vi "Agilent DMM Measure.vi"(7 "Agilent DMM":T2, 8 "error in (no error)":errorcluster, 11 "VISA Resource Name":refnum<visa-resource-name>) -> (0 "error out":errorcluster {"code" format="%.0x"}, 2 "DMM Measurement":T1 caption="This reading is allways in the base units\ni.e. V, A, Ohms, Hz, Sec, etc." format="%#_10f", 3 "dup VISA Resource Name":refnum<visa-resource-name>)   [LabVIEW 2011]
uses:
  TypeDefs/Agilent DMM Instrument Info.ctl
  DMM Measurement.ctl
  TypeDefs/Agilent DMM Trigger Source.ctl
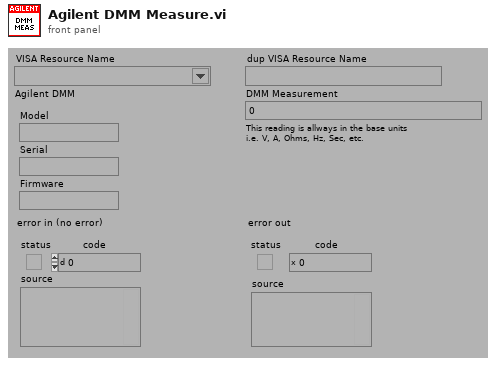
[diagram p1: front panel]
types:
  T1 = typedef "DMM Measurement.ctl" = dbl
  T2 = typedef "Agilent DMM Instrument Info.ctl" = cluster{"Model":string, "Serial":string, "Firmware":string}
  T3 = typedef "Agilent DMM Trigger Source.ctl" = enum16{"Immediate", "Bus", "External"}
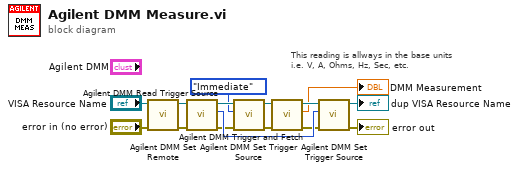
[diagram p0: block diagram]
diagram:
  # "This reading is allways in the base units\ni.e. V, A, Ohms, Hz, Sec, etc."
  n1 = call "Agilent DMM Set Remote.vi"("error in (no error)"="error in (no error)", "VISA Resource Name"="VISA Resource Name") -> ("error out"=w6:errorcluster, "dup VISA Resource Name"=w7:refnum<visa-resource-name>)  [unwired: 8 out]
  n2 = call "Agilent DMM Read Trigger Source.vi"("error in (no error)"=w6, "VISA Resource Name"=w7) -> ("error out"=w2:errorcluster, "Trigger Source"=w13:T3, "dup VISA Resource Name"=w3:refnum<visa-resource-name>)  [unwired: 7 out]
  n3 = call "Agilent DMM Set Trigger Source.vi"("error in (no error)"=w2, "Trigger Source"=Agilent_DMM_Trigger_Source."Immediate", "VISA Resource Name"=w3) -> ("error out"=w5:errorcluster, "dup VISA Resource Name"=w4:refnum<visa-resource-name>)  [unwired: 7 out]
  n4 = call "Agilent DMM Trigger and Fetch.vi"("error in (no error)"=w5, "VISA Resource Name"=w4) -> ("error out"=w12:errorcluster, "Data Reading"=→"DMM Measurement":T1, "dup VISA Resource Name"=w11:refnum<visa-resource-name>)  [unwired: 1 in, 6 out]
  n5 = call "Agilent DMM Set Trigger Source.vi"("error in (no error)"=w12, "Trigger Source"=w13, "VISA Resource Name"=w11) -> ("error out"=→"error out":errorcluster, "dup VISA Resource Name"=→"dup VISA Resource Name":refnum<visa-resource-name>)  [unwired: 7 out]
